vi "Read Frequency.vi"(11 "AM-AM in":refnum<class "AM-AM.lvclass">) -> (2 "Frequency":cluster{"List":dbl[], "Index":i32, "Last":bool}, 3 "AM-AM out":refnum<class "AM-AM.lvclass">)   [LabVIEW 2020, in "AM-AM.lvclass"]
uses:
  AM-AM.lvclass
  AM-AM.lvclass/AM-AM.ctl
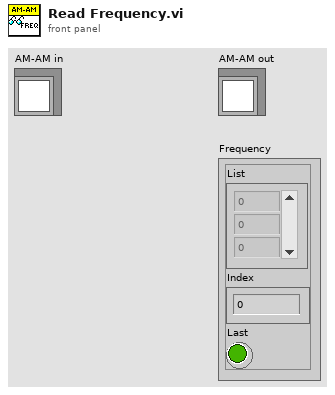
[diagram p1: front panel]
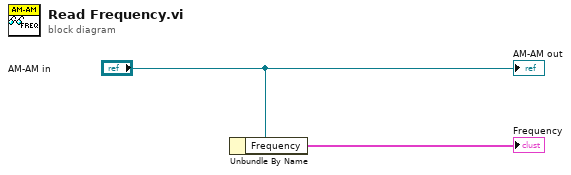
[diagram p0: block diagram]
diagram:
  n1 = Unbundle By Name("AM-AM in") -> ("Frequency"=→"Frequency":cluster{"List":dbl[], "Index":i32, "Last":bool})
  "AM-AM out" <- "AM-AM in"
